vi "Get API.vi"(8 "error in (no error)":errorcluster, 11 "Actor in":refnum<class "Actor.lvclass">) -> (0 "error out":errorcluster, 2 "Actor API":refnum<class "Actor API.lvclass">, 3 "Actor out":refnum<class "Actor.lvclass">)   [LabVIEW 2022 SP3, in "Artifex.lvlib" / "Actor.lvclass"]
uses:
  Actor.lvclass
  Actor Proxy/Actor API.lvclass
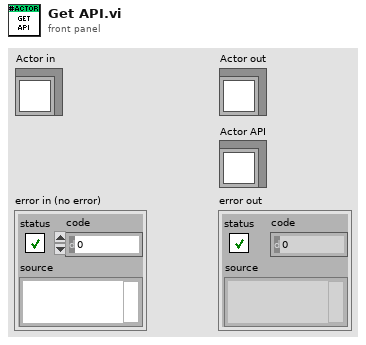
[diagram p1: front panel]
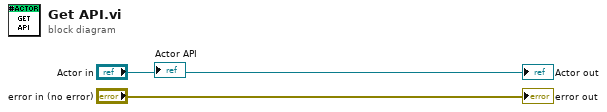
[diagram p0: block diagram]
diagram:
  "error out" <- "error in (no error)"
  "Actor out" <- "Actor in"
